vi "Untitled 4.vi"   [LabVIEW 2016]
uses:
  PublicSubvi/BoolACT.ctl
types:
  T1 = typedef "BoolACT.ctl" = enum16{"Get", "Set"}
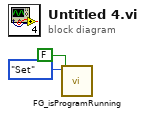
[diagram p0: block diagram]
diagram:
  n1 = call "FG_isProgramRunning"("Value"=FALSE, "ACT"=BoolACT."Set") -> ()  [unwired: 8 in, 2 out]
